vi "Create Wrist Constants.vi"(1 "error in":errorcluster, 2 "localConstantSpreadSheet":string[][](array[string]), 3 "robotID":string) -> (0 "error out":errorcluster)   [LabVIEW 2020]
uses:
  2023 Robot Global Data.vi
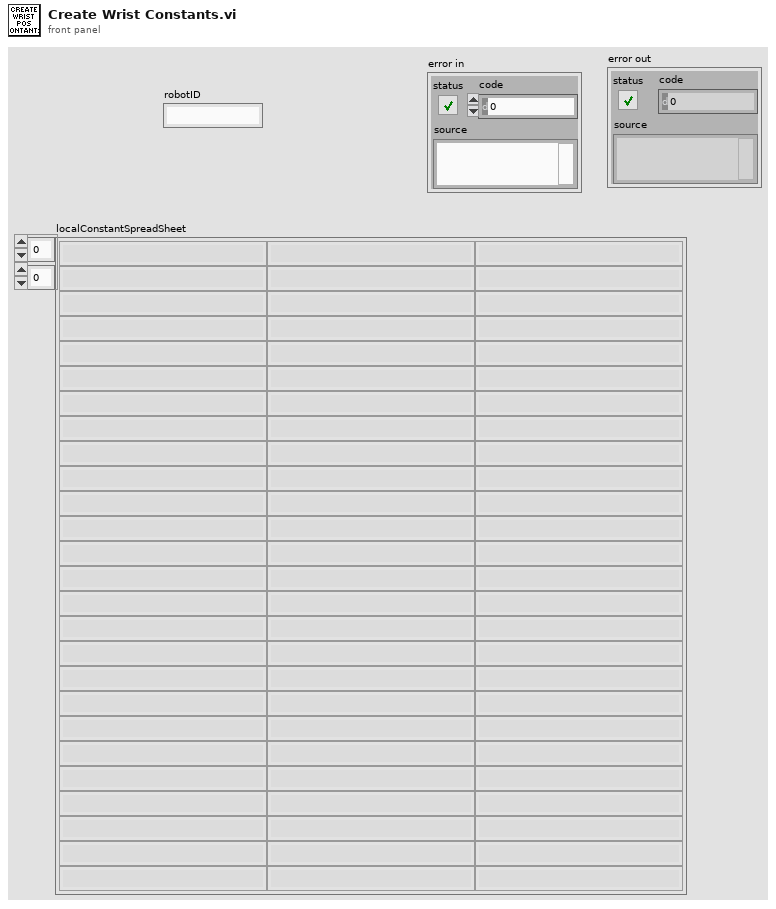
[diagram p1: front panel]
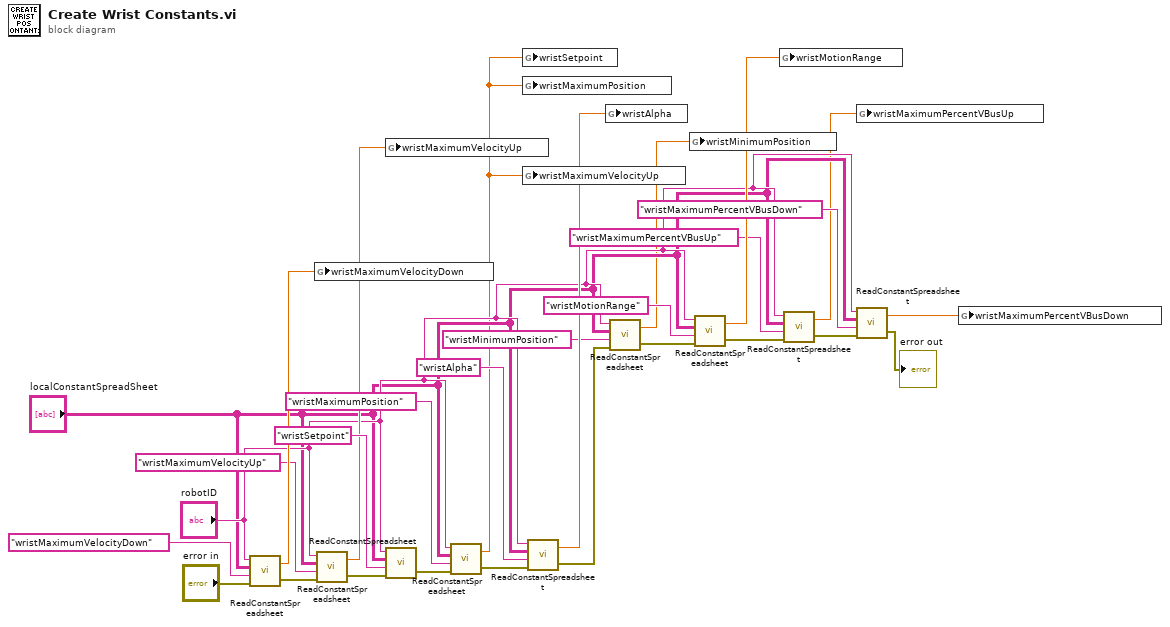
[diagram p0: block diagram]
diagram:
  n1 = call "ReadConstantSpreadsheet.vi"("error in"="error in", "Constant"="wristMaximumVelocityDown", "2023ConstantSpreadSheet"="localConstantSpreadSheet", "Robot ID"="robotID") -> ("error out"=w12:errorcluster, "Constant Value"=w27:dbl)
  n2 = global write "2023 Robot Global Data.vi" "wristMaximumVelocityDown"(w27) -> ()
  n3 = call "ReadConstantSpreadsheet.vi"("error in"=w12, "Constant"="wristMaximumVelocityUp", "2023ConstantSpreadSheet"="localConstantSpreadSheet", "Robot ID"="robotID") -> ("error out"=w11:errorcluster, "Constant Value"=w10:dbl)
  n4 = global write "2023 Robot Global Data.vi" "wristMaximumVelocityUp"(w10) -> ()
  n5 = call "ReadConstantSpreadsheet.vi"("error in"=w11, "Constant"="wristSetpoint", "2023ConstantSpreadSheet"="localConstantSpreadSheet", "Robot ID"="robotID") -> ("error out"=w4:errorcluster)  [unwired: 1 out]
  n6 = call "ReadConstantSpreadsheet.vi"("error in"=w4, "Constant"="wristMaximumPosition", "2023ConstantSpreadSheet"="localConstantSpreadSheet", "Robot ID"="robotID") -> ("error out"=w19:errorcluster, "Constant Value"=w1:dbl)
  n7 = global write "2023 Robot Global Data.vi" "wristSetpoint"(w1) -> ()
  n8 = global write "2023 Robot Global Data.vi" "wristMaximumPosition"(w1) -> ()
  n9 = global write "2023 Robot Global Data.vi" "wristMaximumVelocityUp"(w1) -> ()
  n10 = call "ReadConstantSpreadsheet.vi"("error in"=w19, "Constant"="wristAlpha", "2023ConstantSpreadSheet"="localConstantSpreadSheet", "Robot ID"="robotID") -> ("error out"=w18:errorcluster, "Constant Value"=w25:dbl)
  n11 = global write "2023 Robot Global Data.vi" "wristAlpha"(w25) -> ()
  n12 = call "ReadConstantSpreadsheet.vi"("error in"=w18, "Constant"="wristMinimumPosition", "2023ConstantSpreadSheet"="localConstantSpreadSheet", "Robot ID"="robotID") -> ("error out"=w17:errorcluster, "Constant Value"=w3:dbl)
  n13 = global write "2023 Robot Global Data.vi" "wristMinimumPosition"(w3) -> ()
  n14 = call "ReadConstantSpreadsheet.vi"("error in"=w17, "Constant"="wristMotionRange", "2023ConstantSpreadSheet"="localConstantSpreadSheet", "Robot ID"="robotID") -> ("error out"=w9:errorcluster, "Constant Value"=w29:dbl)
  n15 = global write "2023 Robot Global Data.vi" "wristMotionRange"(w29) -> ()
  n16 = call "ReadConstantSpreadsheet.vi"("error in"=w9, "Constant"="wristMaximumPercentVBusUp", "2023ConstantSpreadSheet"="localConstantSpreadSheet", "Robot ID"="robotID") -> ("error out"=w8:errorcluster, "Constant Value"=w2:dbl)
  n17 = global write "2023 Robot Global Data.vi" "wristMaximumPercentVBusUp"(w2) -> ()
  n18 = call "ReadConstantSpreadsheet.vi"("error in"=w8, "Constant"="wristMaximumPercentVBusDown", "2023ConstantSpreadSheet"="localConstantSpreadSheet", "Robot ID"="robotID") -> ("error out"=→"error out":errorcluster, "Constant Value"=w16:dbl)
  n19 = global write "2023 Robot Global Data.vi" "wristMaximumPercentVBusDown"(w16) -> ()
